vi "Lissajous Graph.vi"() -> ()   [LabVIEW 2012]
uses:
  <vilib>/Analysis/NI_AALBase.lvlib
panel:
  in  "samples":i32=1024 caption="采样"
  in  "Second Curve":dbl=3.0 caption="周期" format="%0.2f"
  in  "First Curve":dbl=4.0 format="%0.2f"
  out "Lissajous  Graph":T1(graph)
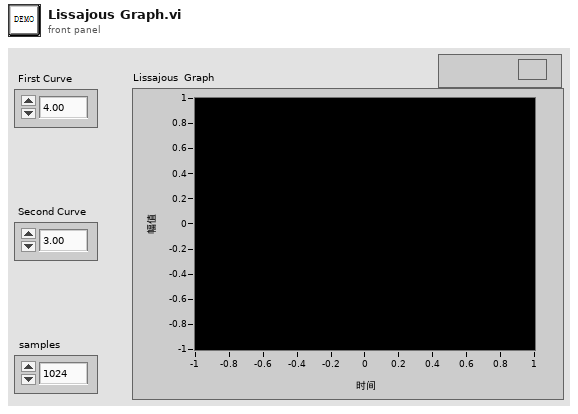
[diagram p1: front panel]
types:
  T1 = cluster{"Sinusoidal Pattern":dbl[], "Sinusoidal Pattern":dbl[]}
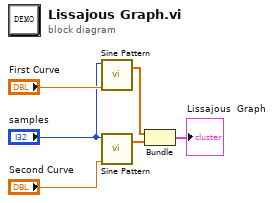
[diagram p0: block diagram]
diagram:
  n1 = call <vilib>:"Sine Pattern.vi"("cycles"="First Curve", "samples"="samples") -> ("Sinusoidal Pattern"=w4:dbl[])  [unwired: 2 in, 1 out]
  n2 = call <vilib>:"Sine Pattern.vi"("cycles"="Second Curve", "samples"="samples") -> ("Sinusoidal Pattern"=w3:dbl[])  [unwired: 2 in, 1 out]
  n3 = Bundle("Sinusoidal Pattern"=w4, "Sinusoidal Pattern"=w3) -> (→"Lissajous  Graph":T1)  [unwired: 1 in]
